vi "fit function -1 over T.vi"(3 "output control":T1, 4 "data":T2, 5 "X":dbl[](array[numeric]), 6 "a":dbl[](array[numeric])) -> (0 "error out":errorcluster, 1 "f'(X,a)":dbl[][](array[numeric]), 2 "f(X,a)":dbl[](array[numeric]))   [LabVIEW 2014]
doc: "This template is the starting point for creating a model function to be passed to the Nonlinear Curve Fit.vi."
uses:
  <vilib>/gmath/NumericalOptimization/objective function data.ctl
  <vilib>/gmath/NumericalOptimization/LM_output select.ctl
  <vilib>/gmath/NI_Gmath.lvlib
panel:
  in  "power":dbl=1.0
  in  "fit":enum16{"other", "3par", "5par"}(ring)=enum."3par"
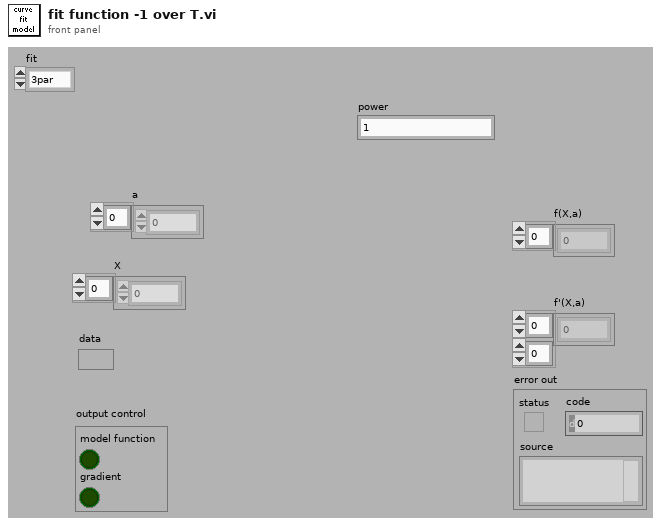
[diagram p1: front panel]
types:
  T1 = typedef "NI_Gmath.lvlib/LM_output select.ctl" = cluster{"model function":bool, "gradient":bool}
  T2 = typedef "NI_Gmath.lvlib/objective function data.ctl" = variant
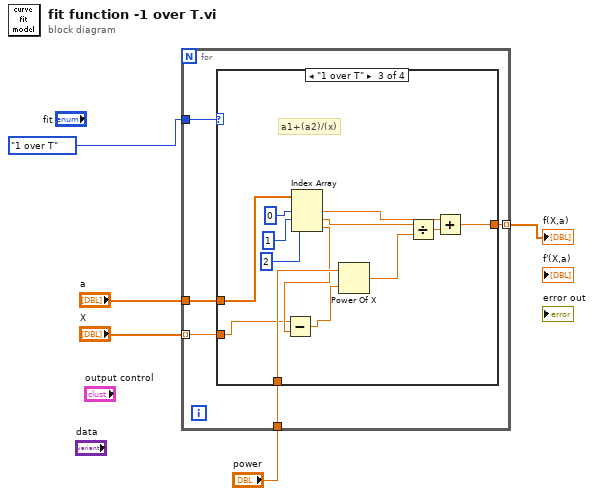
[diagram p0: block diagram]
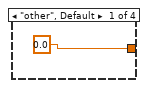
[diagram p2: hidden frame]
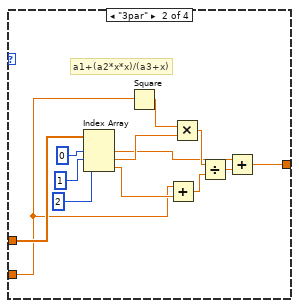
[diagram p3: hidden frame]
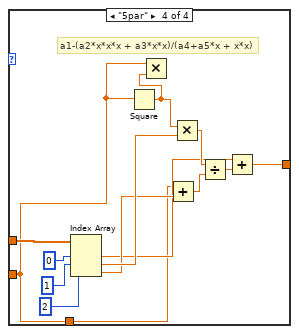
[diagram p4: hidden frame]
diagram:
  n1 = for {
    tunnel: "a" -> [w10]
    tunnel: "X" -> [w8] mode=indexing
    tunnel: [w9] -> w3 mode=indexing
    tunnel: enum16{"other", "3par", "5par", "1 over T"}."1 over T" ("action") -> [w7]
    tunnel: "power" -> [w6]
    n2 = case shown="\"1 over T\"" w7 {
      tunnel: w10 -> [_ w24 w37 w50]
      tunnel: [0.0 w14 w32 w40] -> w9
      tunnel: w8 -> [_ w13 w26 w39]
      tunnel: w6 -> [_ _ w30 _]
      frame "other", Default {
      }
      frame "3par" {
        # "a1+(a2*x*x)/(a3+x)"
        n3 = Index Array(array=w24, index #1=0 ("index"), index #2=1 ("index"), index #3=2 ("index")) -> (element #1=w16:dbl, element #2=w20:dbl, element #3=w19:dbl)
        n4 = Square(x=w13) -> (x^2=w12:dbl)
        n5 = Add(x=w13, y=w19) -> (x+y=w17:dbl)
        n6 = Multiply(x=w12, y=w20) -> (x*y=w18:dbl)
        n7 = Divide(x=w18, y=w17) -> (x/y=w15:dbl)
        n8 = Add(x=w16, y=w15) -> (x+y=w14:dbl)
      }
      frame "1 over T" {
        # "a1+(a2)/(x)"
        n9 = Index Array(array=w37, index #1=0 ("index"), index #2=1 ("index"), index #3=2 ("index")) -> (element #1=w34:dbl, element #2=w31:dbl, element #3=w27:dbl)
        n10 = Subtract(x=w26, y=w27) -> (x-y=w25:dbl)
        n11 = Power Of X(1:w25, 2:w30) -> (0:w29:dbl)
        n12 = Divide(x=w31, y=w29) -> (x/y=w33:dbl)
        n13 = Add(x=w34, y=w33) -> (x+y=w32:dbl)
      }
      frame "5par" {
        # "a1-(a2*x*x*x + a3*x*x)/(a4+a5*x + x*x)"
        n14 = Index Array(array=w50, index #1=0 ("index"), index #2=1 ("index"), index #3=2 ("index")) -> (element #1=w42:dbl, element #2=w46:dbl, element #3=w45:dbl)
        n15 = Square(x=w39) -> (x^2=w38:dbl)
        n16 = Multiply(x=w39, y=w38) -> ()  [unwired: 1 out]
        n17 = Add(x=w39, y=w45) -> (x+y=w43:dbl)
        n18 = Multiply(x=w38, y=w46) -> (x*y=w44:dbl)
        n19 = Divide(x=w44, y=w43) -> (x/y=w41:dbl)
        n20 = Add(x=w42, y=w41) -> (x+y=w40:dbl)
      }
    }
  }
  "f(X,a)" <- w3
